vi "usrp set tx lo freq.vi"(6 "coerced_freq_out":dbl, 7 "chan":u64, 8 "error in (no error)":errorcluster, 9 "name":string, 10 "freq":dbl, 11 "h":u64) -> (0 "error out":errorcluster, 3 "function return":u32(ring), 4 "coerced_freq_out out":dbl)   [LabVIEW 2023, in "uhd.lvlib"]
doc: "UHD_API uhd_error uhd_usrp_set_tx_lo_freq(uhd_usrp_handle h,\n double freq,\n const char* name,\n size_t chan,\n double* coerced_freq_out);"
uses:
  <userlib>/uhd/uhd.lvlib
  <userlib>/uhd/uhd.dll
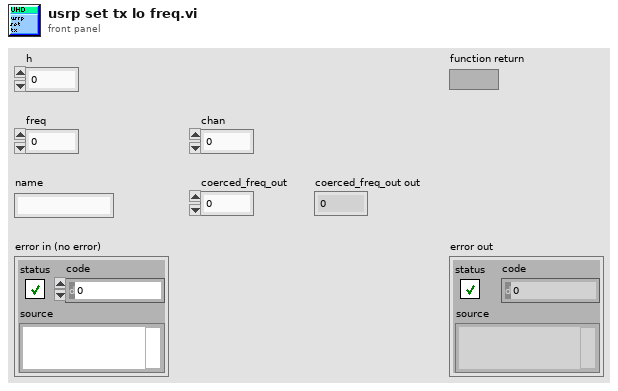
[diagram p1: front panel]
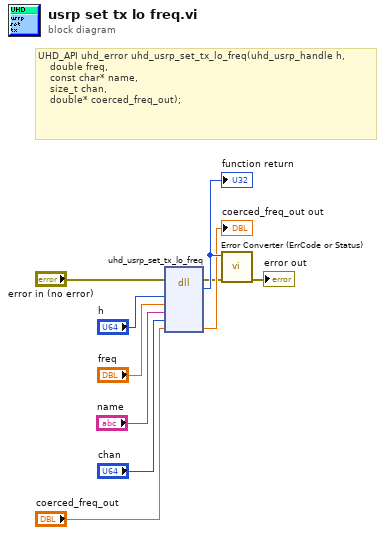
[diagram p0: block diagram]
diagram:
  # "UHD_API uhd_error uhd_usrp_set_tx_lo_freq(uhd_usrp_handle h,\n    double freq,\n    const char* name,\n    size_t chan,\n    double* coerced_freq_out);"
  n1 = dll-call lib="C:/Program Files/National Instruments/LabVIEW 2023/user.lib/uhd/uhd.*" fn="uhd_usrp_set_tx_lo_freq"(error in="error in (no error)", "h"="h", "freq"="freq", "name"="name", "chan"="chan", "coerced_freq_out"="coerced_freq_out") -> (error out=w2:errorcluster, w10:u32, "coerced_freq_out"=→"coerced_freq_out out":dbl)  [unwired: 6 in, 1 out]
  "function return" <- w10
  n2 = call <userlib>:"Error Converter (ErrCode or Status).vi"("error in (no error)"=w2, "error code"=w10) -> ("error out"=→"error out":errorcluster)  [unwired: 9 in]
